vi "Reentrant Method Proxy.vi"(8 "error in (no error)":errorcluster, 10 "Numeric in":dbl, 11 "Test Interface Mock in":refnum<class "Test Interface Mock.lvclass">) -> (0 "error out":errorcluster, 3 "Test Interface Mock out":refnum<class "Test Interface Mock.lvclass">)   [LabVIEW 2020, in "Test Interface Mock.lvclass"]
uses:
  Test Interface Mock.lvclass
  C:/git/astemes-lmock/sandbox/Mock/Mock.lvclass
  Mock/Mock.lvclass/Mock.ctl
  Call/Create.vi
  Expectation/Expectation.lvclass
  Mock/Mock.lvclass
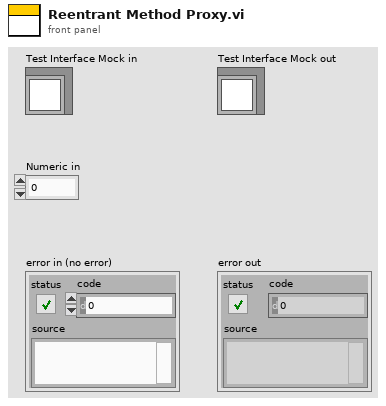
[diagram p1: front panel]
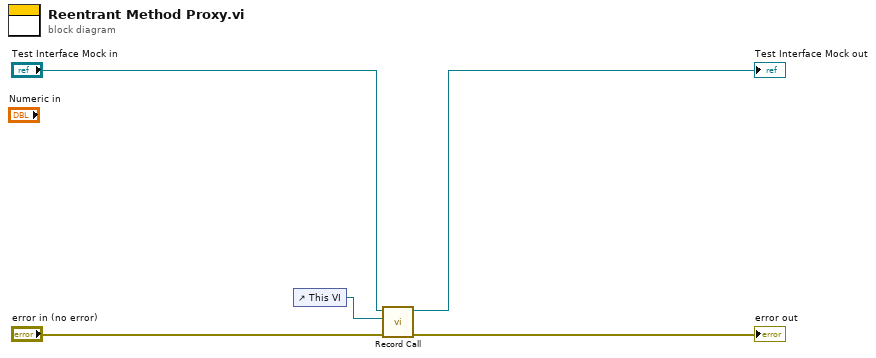
[diagram p0: block diagram]
diagram:
  n1 = control-ref of="This VI"() -> (w1:refnum<vi>)
  n2 = call "Record Call.vi"("error in (no error)"="error in (no error)", "This VI"=w1, "Mock In"="Test Interface Mock in") -> ("error out"=→"error out":errorcluster, "Mock Out"=→"Test Interface Mock out":refnum<class "Test Interface Mock.lvclass">)  [unwired: 7 in]
